vi "Blutooth.vi"() -> ()   [LabVIEW 2023]
uses:
  <vilib>/Utility/error.llb/Trim Whitespace One-Sided.vi
  <vilib>/Instr/_visa.llb/VISA Configure Serial Port (Instr).vi
panel:
  out "Humidity":dbl(slide) scale=0.0..100.0
  out "Temperature":dbl(slide) scale=0.0..100.0
  in  "Boolean 3":bool
  in  "Boolean 2":bool
  in  "Boolean":bool
  in  "stop":bool
  out "read buffer":string
  in  "VISA resource name":refnum<visa-resource-name>
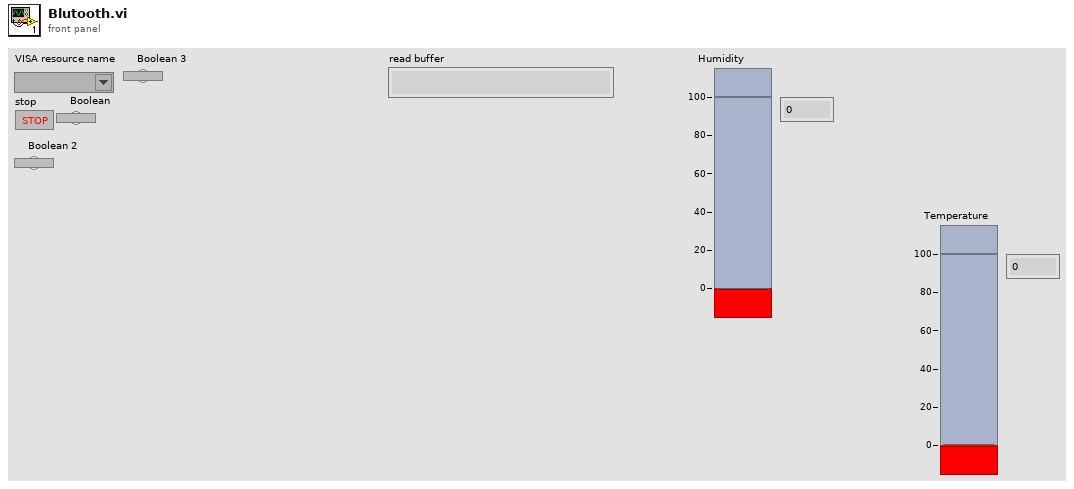
[diagram p1: front panel]
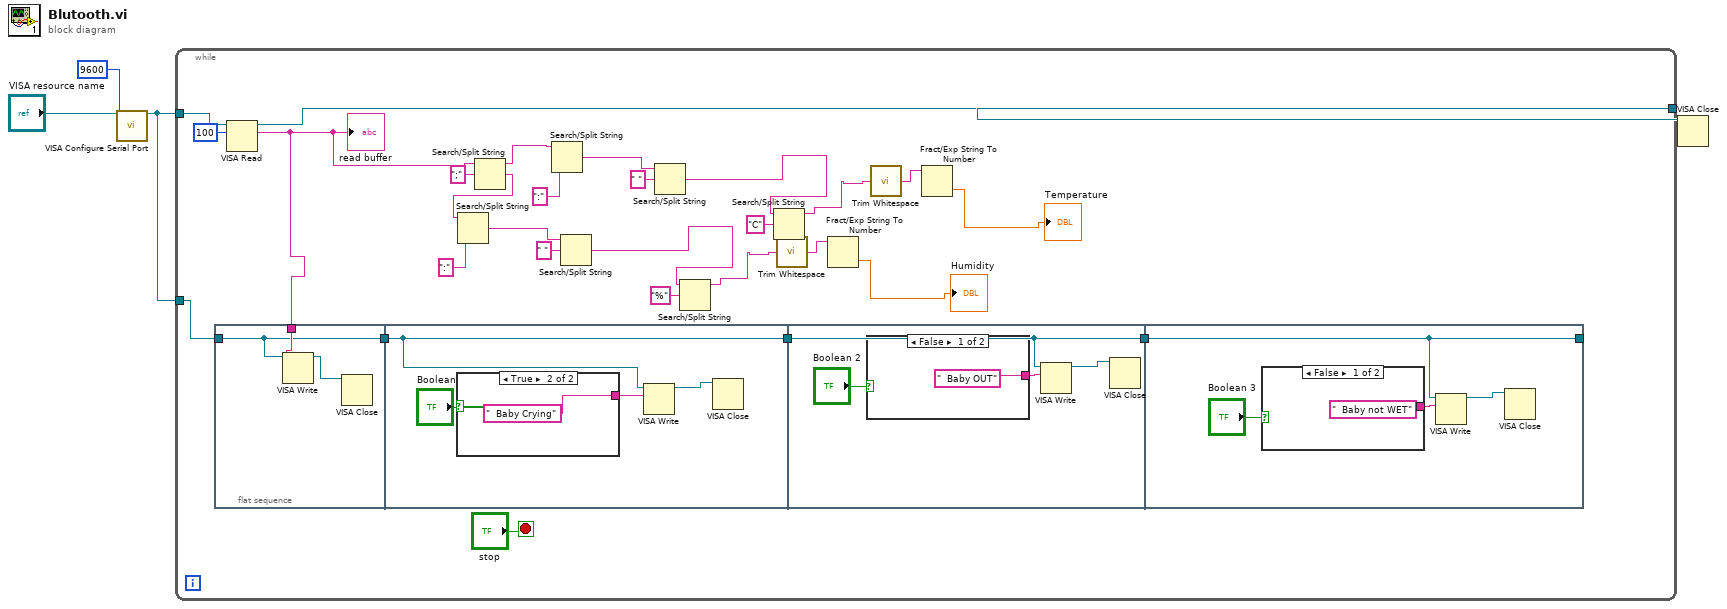
[diagram p0: block diagram]
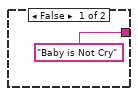
[diagram p2: hidden frame]
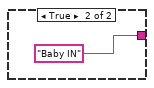
[diagram p3: hidden frame]
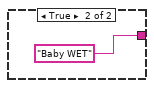
[diagram p4: hidden frame]
diagram:
  n1 = call-poly "VISA Configure Serial Port"("VISA resource name"="VISA resource name", "baud rate (9600)"=u32 9600) -> ("VISA resource name out"=w1:refnum<visa-resource-name>)  [unwired: 12 in, 1 out]
  n2 = while {
    tunnel: w1 -> [w32]
    tunnel: [w29] -> w2
    tunnel: w1 -> [w28]
    stop <- "stop" stop-if-true
    n3 = flat-sequence {
      tunnel: w14 -> [w35]
      tunnel: w28 -> [w34]
      tunnel: [w34] -> w27
      tunnel: w27 -> [w37]
      tunnel: [w37] -> w26
      tunnel: w26 -> [w42]
      tunnel: [w42] -> w25
      tunnel: [w48] -> _
      tunnel: w25 -> [w48]
      frame #0 {
        n4 = VISA Write(VISA resource name=w34, write buffer=w35) -> (VISA resource name out=w33:refnum<visa-resource-name>)  [unwired: 1 in, 2 out]
        n5 = VISA Close(VISA resource name=w33) -> ()  [unwired: 1 in, 1 out]
      }
      frame #1 {
        n6 = case shown="True" "Boolean" {
          tunnel: ["Baby is Not Cry" "  Baby Crying"] -> w38
          frame False {
          }
          frame True {
          }
        }
        n7 = VISA Write(VISA resource name=w37, write buffer=w38) -> (VISA resource name out=w36:refnum<visa-resource-name>)  [unwired: 1 in, 2 out]
        n8 = VISA Close(VISA resource name=w36) -> ()  [unwired: 1 in, 1 out]
      }
      frame #2 {
        n9 = case shown="False" "Boolean 2" {
          tunnel: ["  Baby OUT" "Baby IN"] -> w44
          frame False {
          }
          frame True {
          }
        }
        n10 = VISA Write(VISA resource name=w42, write buffer=w44) -> (VISA resource name out=w43:refnum<visa-resource-name>)  [unwired: 1 in, 2 out]
        n11 = VISA Close(VISA resource name=w43) -> ()  [unwired: 1 in, 1 out]
      }
      frame #3 {
        n12 = case shown="False" "Boolean 3" {
          tunnel: ["  Baby not WET" "Baby WET"] -> w50
          frame False {
          }
          frame True {
          }
        }
        n13 = VISA Write(VISA resource name=w48, write buffer=w50) -> (VISA resource name out=w49:refnum<visa-resource-name>)  [unwired: 1 in, 2 out]
        n14 = VISA Close(VISA resource name=w49) -> ()  [unwired: 1 in, 1 out]
      }
    }
    n15 = VISA Read(VISA resource name=w32, byte count=u32 100) -> (VISA resource name out=w29:refnum<visa-resource-name>, read buffer=w14:string)  [unwired: 1 in, 2 out]
    "read buffer" <- w14
    n16 = Search/Split String(string=w14, search string/char (-)=";") -> (substring before match=w23:string, match + rest of string=w5:string)  [unwired: 1 in, 1 out]
    n17 = Search/Split String(string=w5, search string/char (-)=":") -> (match + rest of string=w11:string)  [unwired: 1 in, 2 out]
    n18 = Search/Split String(string=w23, search string/char (-)=":") -> (match + rest of string=w20:string)  [unwired: 1 in, 2 out]
    n19 = Search/Split String(string=w11, search string/char (-)=" ") -> (match + rest of string=w9:string)  [unwired: 1 in, 2 out]
    n20 = Search/Split String(string=w20, search string/char (-)=" ") -> (match + rest of string=w18:string)  [unwired: 1 in, 2 out]
    n21 = Search/Split String(string=w9, search string/char (-)="%") -> (substring before match=w8:string)  [unwired: 1 in, 2 out]
    n22 = Search/Split String(string=w18, search string/char (-)="C") -> (substring before match=w17:string)  [unwired: 1 in, 2 out]
    n23 = call <vilib>:"Trim Whitespace.vi"("string"=w8) -> ("trimmed string"=w7:string)  [unwired: 1 in]
    n24 = Fract/Exp String To Number(string=w7) -> (number=→"Humidity":dbl)  [unwired: 3 in, 1 out]
    n25 = call <vilib>:"Trim Whitespace.vi"("string"=w17) -> ("trimmed string"=w16:string)  [unwired: 1 in]
    n26 = Fract/Exp String To Number(string=w16) -> (number=→"Temperature":dbl)  [unwired: 3 in, 1 out]
  }
  n27 = VISA Close(VISA resource name=w2) -> ()  [unwired: 1 in, 1 out]
